vi "Get_Preinitialized_Images-1.vi"(5 "error IN":errorcluster, 7 "[IN] Number of event":i8, 8 "[IN] Images Array":T1[](array[typedef])) -> (0 "error OUT":errorcluster, 1 "[OUT] Processed Image #2":T1, 2 "[OUT] Processed Image #1":T1, 3 "[OUT] Source Image #2":T1, 4 "[OUT] Source Image #1":T1)   [LabVIEW 2013]
doc: "Get references to images from generated array"
uses:
  <vilib>/vision/Image Controls.llb/IMAQ Image.ctl
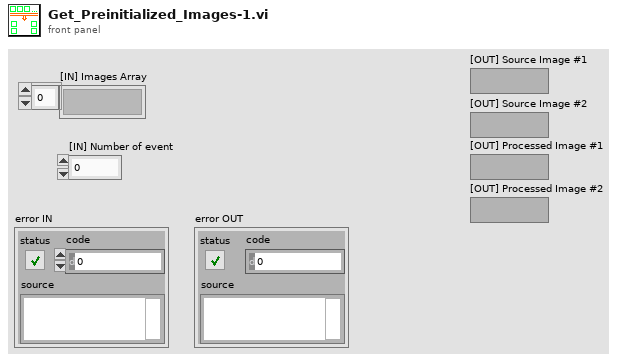
[diagram p1: front panel]
types:
  T1 = typedef "IMAQ Image.ctl" = refnum<image>
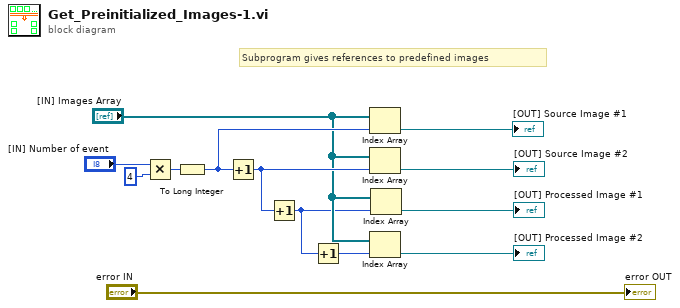
[diagram p0: block diagram]
diagram:
  # "Subprogram gives references to predefined images"
  n1 = Multiply(x="[IN] Number of event", y=i8 4) -> (x*y=w11:i8)
  n2 = To Long Integer(number=w11) -> (32bit integer=w7:i32)
  n3 = Increment(x=w7) -> (x+1=w6:i32)
  n4 = Increment(x=w6) -> (x+1=w2:i32)
  n5 = Increment(x=w2) -> (x+1=w1:i32)
  n6 = Index Array(array="[IN] Images Array", index=w7) -> (element=→"[OUT] Source Image #1":T1)
  n7 = Index Array(array="[IN] Images Array", index=w6) -> (element=→"[OUT] Source Image #2":T1)
  n8 = Index Array(array="[IN] Images Array", index=w1) -> (element=→"[OUT] Processed Image #2":T1)
  n9 = Index Array(array="[IN] Images Array", index=w2) -> (element=→"[OUT] Processed Image #1":T1)
  "error OUT" <- "error IN"
